vi "OSSP_Problem_Attributes_Getter.vi"(8 "error in (no error)":errorcluster, 11 "OSSP_Problem in":refnum<class "OSSP_Problem.lvclass">) -> (0 "error out":errorcluster, 1 "Machines":u16[][](array[numeric]), 2 "Processing Times":u16[][](array[numeric]), 3 "OSSP_Problem out":refnum<class "OSSP_Problem.lvclass">, 4 "Falttened Proceesing Times":u16[](array[numeric]), 5 "Dimension":i32)   [LabVIEW 2013, in "OSSP_Problem.lvclass"]
uses:
  OSSP_Problem.lvclass
  OSSP_Problem.lvclass/OSSP_Problem.ctl
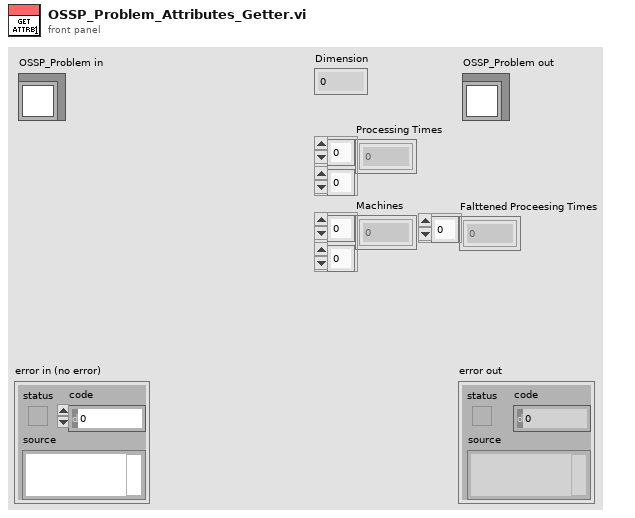
[diagram p1: front panel]
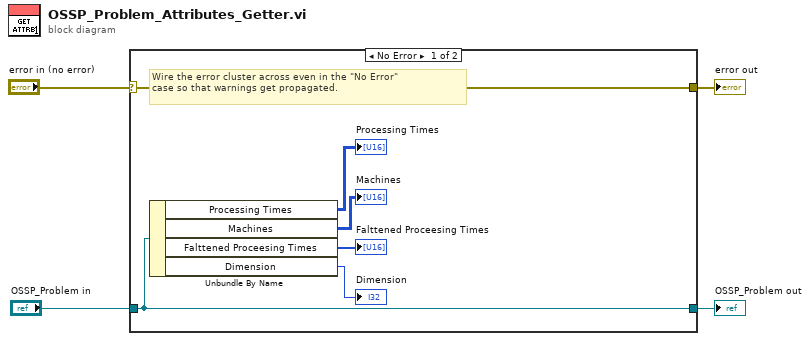
[diagram p0: block diagram]
diagram:
  n1 = case shown="No Error" "error in (no error)" {
    selector: "error in (no error)" -> [w10 w12]
    tunnel: [w10 w12] -> w3
    tunnel: [w9 w11] -> w1
    tunnel: "OSSP_Problem in" -> [w9 w11]
    frame No Error {
      # "Wire the error cluster across even in the \"No Error\"\ncase so that warnings get propagated."
      n2 = Unbundle By Name(w9) -> ("Processing Times"=→"Processing Times":u16[][], "Machines"=→"Machines":u16[][], "Falttened Proceesing Times"=→"Falttened Proceesing Times":u16[], "Dimension"=→"Dimension":i32)
    }
    frame Error {
    }
  }
  "error out" <- w3
  "OSSP_Problem out" <- w1
